vi "get_subsystem_queue.vi"(6 "Line #":i32, 9 "Line in":string, 11 "Subsystem in":string) -> ()   [LabVIEW 2017, in "labview-standard-library.lvlib" / "automode-scripting.lvlib"]
uses:
  automode-scripting.lvlib
  type-defs/command_line_info.ctl
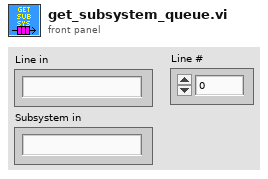
[diagram p1: front panel]
types:
  T1 = typedef "labview-standard-library.lvlib/automode-scripting.lvlib/command_line_info.ctl" = cluster{"Line text":string, "Line #":i32}
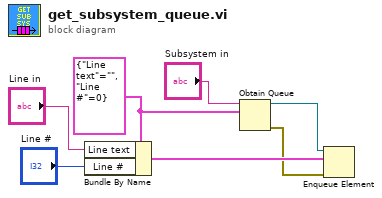
[diagram p0: block diagram]
diagram:
  w2 = T1 {"Line text"="", "Line #"=0}
  n1 = Bundle By Name(cluster=w2, "Line text"="Line in", "Line #"="Line #") -> (w6:T1)
  n2 = Obtain Queue(name (unnamed)="Subsystem in", element data type=w2) -> (queue out=w3:refnum<queue>, error out=w4:errorcluster)  [unwired: 3 in, 1 out]
  n3 = Enqueue Element(queue=w3, element=w6, error in (no error)=w4) -> ()  [unwired: 1 in, 3 out]
